vi "Time_Date_Data from timestamp.vi"(8 "error in (no error)":errorcluster, 11 "time stamp in":timestamp) -> (0 "error out":errorcluster, 1 "WeekYearCode":string, 2 "UTC ISO 8601":string, 3 "time stamp":timestamp format="%<%H:%M:%S\n%d/%m/%Y>T", 5 "date time rec UTC":T1, 6 "AM_or_PM?":string, 7 "time_string_underscores":string, 9 "date time rec LOCAL":T1, 10 "date_time_string_underscores":string)   [LabVIEW 2013]
uses:
  <vilib>/Utility/miscctls.llb/LVDateTimeRec.ctl
panel:
  in  "Serial Number":string
  out "BTW WWYYSN":string
  # "YYYYMMDDThhmmssZ"
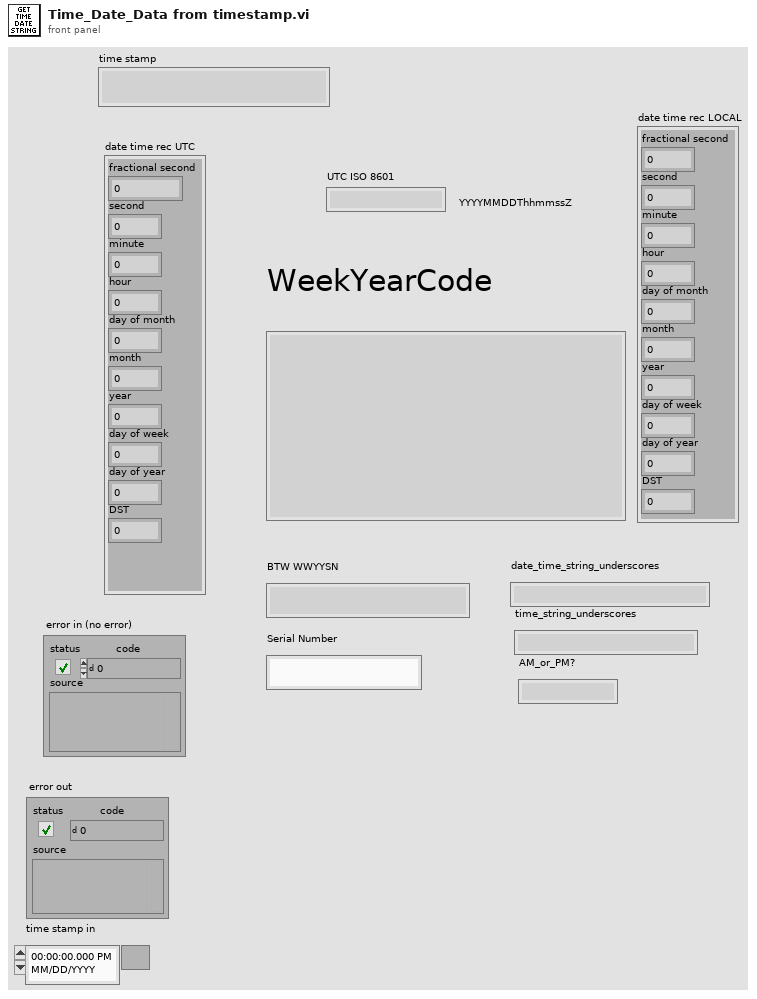
[diagram p1: front panel]
types:
  T1 = typedef "LVDateTimeRec.ctl" = cluster{"fractional second":dbl, "second":i32, "minute":i32, "hour":i32, "day of month":i32, "month":i32, "year":i32, "day of week":i32, "day of year":i32, "DST":i32}
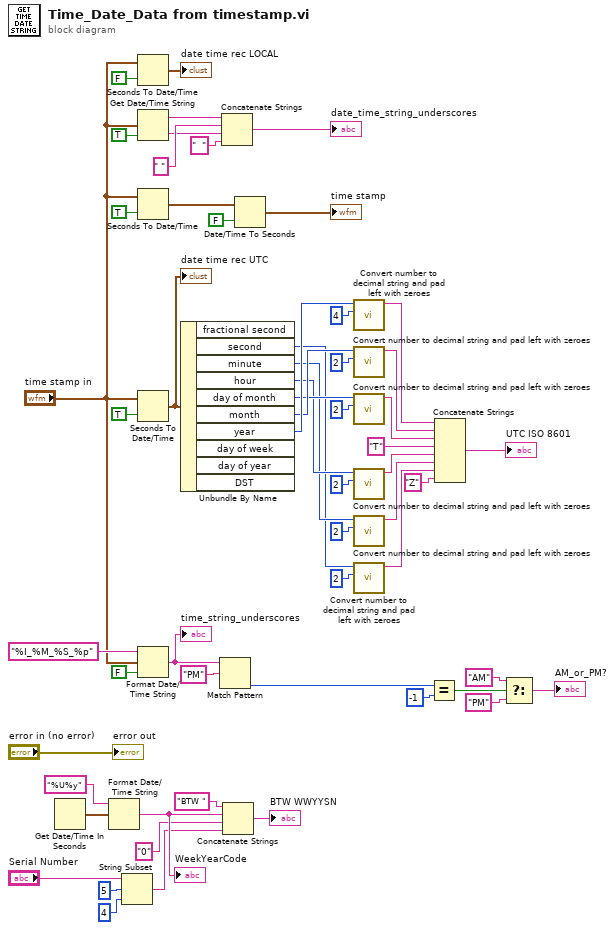
[diagram p0: block diagram]
diagram:
  n1 = Get Date/Time In Seconds() -> (seconds since 1Jan1904=w49:timestamp)
  n2 = Format Date/Time String(time format string (%c)="%U%y", seconds (now)=w49) -> (date/time string=w46:string)  [unwired: 1 in]
  "WeekYearCode" <- w46
  n3 = String Subset(string="Serial Number", offset (0)=5, length (rest)=4 ("length (rest)")) -> (substring=w42:string)
  n4 = Seconds To Date/Time(time stamp (now)="time stamp in", to UTC (F)=FALSE) -> (date time rec=→"date time rec LOCAL":T1)
  n5 = Get Date/Time String(seconds (now)="time stamp in", want seconds? (F)=TRUE) -> (date string=w6:string, time string=w4:string)  [unwired: 1 in]
  n6 = Seconds To Date/Time(time stamp (now)="time stamp in", to UTC (F)=TRUE) -> (date time rec=w55:T1)
  n7 = Seconds To Date/Time(time stamp (now)="time stamp in", to UTC (F)=TRUE) -> (date time rec=w51:T1)
  "date time rec UTC" <- w51
  n8 = Format Date/Time String(time format string (%c)="%I_%M_%S_%p", seconds (now)="time stamp in", UTC format=FALSE) -> (date/time string=w17:string)
  "time_string_underscores" <- w17
  n9 = Unbundle By Name(w51) -> ("second"=w29:i32, "minute"=w31:i32, "hour"=w33:i32, "day of month"=w35:i32, "month"=w37:i32, "year"=w39:i32)  [unwired: 4 out]
  n10 = Match Pattern(string=w17, regular expression="PM") -> (offset past match=w15:i32)  [unwired: 1 in, 3 out]
  n11 = Concatenate Strings(w6, " " ("string"), w4, "  " ("string")) -> (→"date_time_string_underscores":string)
  n12 = Concatenate Strings("BTW " ("string"), w46, "0" ("string"), w42) -> (→"BTW WWYYSN":string)
  n13 = Date/Time To Seconds(1:FALSE ("to UTC (F)"), 2:w55) -> (0:→"time stamp":timestamp)
  n14 = call "Convert number to decimal string and pad left with zeroes.vi"("Width"=u32 4, "number"=w39) -> ("result string"=w27:string)  [unwired: 9 in]
  n15 = call "Convert number to decimal string and pad left with zeroes.vi"("Width"=u32 2, "number"=w37) -> ("result string"=w26:string)  [unwired: 9 in]
  n16 = call "Convert number to decimal string and pad left with zeroes.vi"("Width"=u32 2, "number"=w35) -> ("result string"=w25:string)  [unwired: 9 in]
  n17 = call "Convert number to decimal string and pad left with zeroes.vi"("Width"=u32 2, "number"=w33) -> ("result string"=w23:string)  [unwired: 9 in]
  n18 = call "Convert number to decimal string and pad left with zeroes.vi"("Width"=i16 2 ("width (-)"), "number"=w31) -> ("result string"=w22:string)  [unwired: 9 in]
  n19 = call "Convert number to decimal string and pad left with zeroes.vi"("Width"=i16 2 ("width (-)"), "number"=w29) -> ("result string"=w21:string)  [unwired: 9 in]
  n20 = Equal?(x=w15, y=-1) -> (x = y?=w13:bool)
  n21 = Concatenate Strings(w27, w26, w25, "T" ("string"), w23, w22, w21, "Z" ("string")) -> (→"UTC ISO 8601":string)
  n22 = Select(t="AM" ("regular expression"), s=w13, f="PM" ("regular expression")) -> (s? t:f=→"AM_or_PM?":string)
  "error out" <- "error in (no error)"
